vi "Variable Parser.vi"(11 "Formula":string) -> (3 "Variables":string[](array[string]))   [LabVIEW 2019]
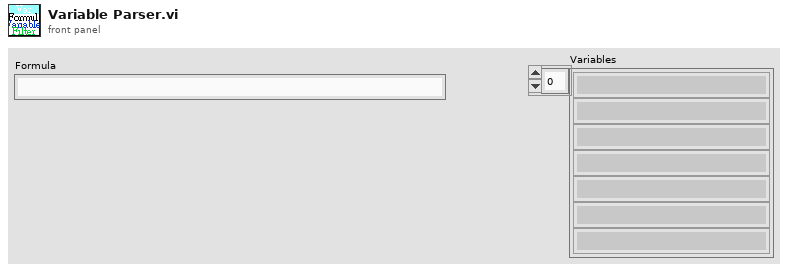
[diagram p1: front panel]
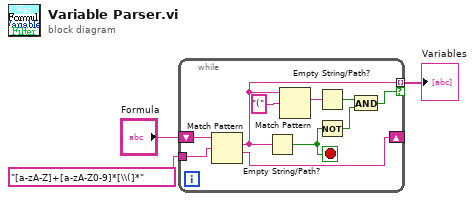
[diagram p0: block diagram]
diagram:
  n1 = while {
    tunnel: "[a-zA-Z]+[a-zA-Z0-9]*[\\(]*" ("regular expression") -> [w12]
    tunnel: [w9] -> w1 mode=indexing if=w5
    shift-right: [w10] -> _
    shift-left: "Formula" -> [w13]
    stop <- w11 stop-if-true
    n2 = Match Pattern(string=w13, regular expression=w12) -> (match substring=w9:string, after substring=w10:string)  [unwired: 1 in, 2 out]
    n3 = Empty String/Path?(string/path=w9) -> (empty?=w11:bool)
    n4 = Match Pattern(string=w9, regular expression="(") -> (match substring=w7:string)  [unwired: 1 in, 3 out]
    n5 = Empty String/Path?(string/path=w7) -> (empty?=w4:bool)
    n6 = Not(x=w11) -> (.not. x?=w6:bool)
    n7 = And(x=w4, y=w6) -> (x .and. y?=w5:bool)
  }
  "Variables" <- w1
